vi "1.8.0 Mutation.vi"(8 "error in":errorcluster, 11 "Device Ref in":T1 format="%.0x") -> (0 "error out":errorcluster, 3 "Device Ref out":T1 format="%.0x")   [LabVIEW 2017, in "Ballard Arinc-429 System Explorer.lvlib"]
uses:
  Ballard Arinc-429 System Explorer.lvlib
  <vilib>/NI Veristand/Custom Device API/Custom Device Item Ref.ctl
  <vilib>/NI Veristand/Custom Device Tools/Custom Device Utility Library/Custom Device Utility Library.lvlib
  <vilib>/NI Veristand/Custom Device Tools/Custom Device Utility Library/NI VeriStand - Search for Item by Name.vi
  Shared/Controls and Global/Global.vi
  Shared/Ballard Arinc-429 Shared.lvlib
  <vilib>/NI Veristand/Custom Device API/Custom Device API.lvlib
  NationalInstruments.VeriStand.SystemStorage
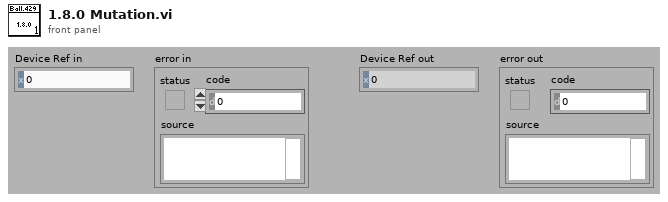
[diagram p1: front panel]
types:
  T1 = typedef "Custom Device API.lvlib/Custom Device Item Ref.ctl" = u64
  T2 = typedef "Custom Device API.lvlib/Custom Device Pointer.ctl" = refnum<k24>
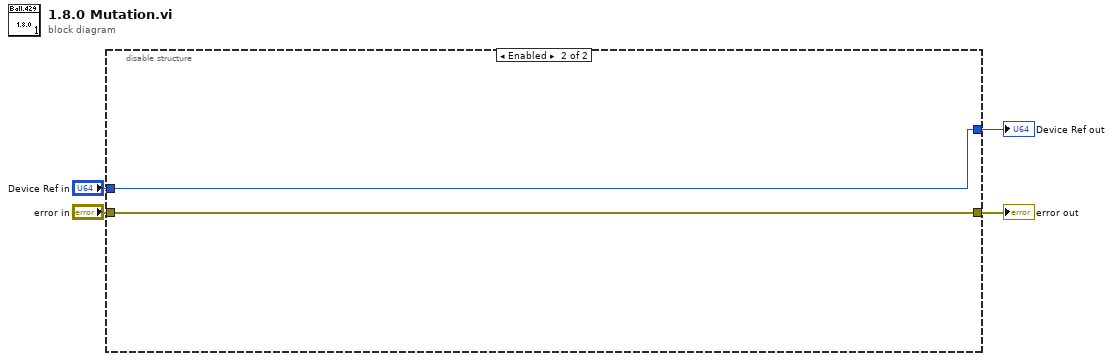
[diagram p0: block diagram]
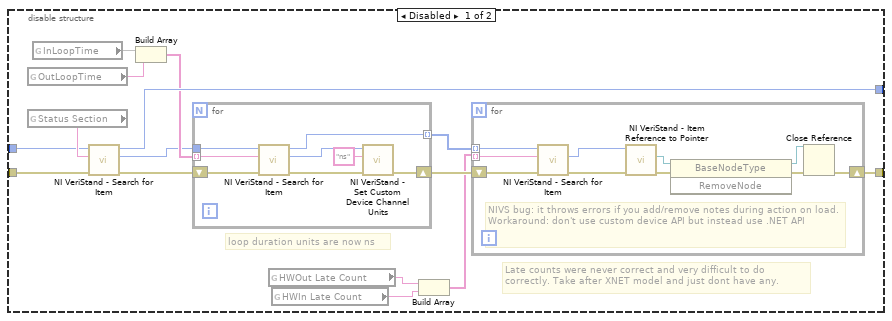
[diagram p2: hidden frame]
diagram:
  n1 = disable-structure shown="Enabled" {
    disable-tunnel: [w19 w39] -> w4
    disable-tunnel: "Device Ref in" -> [w12 w39]
    disable-tunnel: "error in" -> [w11 w38]
    disable-tunnel: [w5 w38] -> w1
    frame Disabled {
      # "Late counts were never correct and very difficult to do correctly. Take after XNET model and just dont have any."
      # "loop duration units are now ns"
      n2 = global read "Global.vi" "OutLoopTime"() -> (w17:string)
      n3 = global read "Global.vi" "Status Section"() -> (w13:string)
      n4 = global read "Global.vi" "InLoopTime"() -> (w16)
      n5 = call-poly <vilib>:"NI VeriStand - Search for Item.vi"("error in"=w11, "Item Name"=w13, "Section Ref in"=w12) -> ("error out"=w15:errorcluster, "Item Ref"=w14:T1, "Section Ref out"=w19:T1)  [unwired: 5 in, 1 out]
      n6 = Build Array(w16, w17) -> (w18:string[])
      n7 = for {
        tunnel: w14 -> [w37]
        shift-right: [w33] -> w9
        shift-left: w15 -> [w36]
        tunnel: w18 -> [w35] mode=indexing
        tunnel: [w30] -> w10 mode=indexing
        n8 = call-poly <vilib>:"NI VeriStand - Search for Item.vi"("error in"=w36, "Item Name"=w35, "Section Ref in"=w37) -> ("error out"=w34:errorcluster, "Item Ref"=w32:T1, "Section Ref out"=w30:T1)  [unwired: 5 in, 1 out]
        n9 = call <vilib>:"NI VeriStand - Set Custom Device Channel Units.vi"("error in (no error)"=w34, "Units"="ns", "Channel Ref in"=w32) -> ("error out"=w33:errorcluster)  [unwired: 7 in, 1 out]
      }
      n10 = global read "Global.vi" "HWOut Late Count"() -> (w8:string)
      n11 = global read "Global.vi" "HWIn Late Count"() -> (w7:string)
      n12 = Build Array(w8, w7) -> (w6:string[])
      n13 = for {
        tunnel: w10 -> [w29] mode=indexing
        shift-right: [w21] -> w5
        shift-left: w9 -> [w28]
        tunnel: w6 -> [w27] mode=indexing
        # "NIVS bug: it throws errors if you add/remove notes during action on load. Workaround: don't use custom device API but instead use .NET API"
        n14 = call-poly <vilib>:"NI VeriStand - Search for Item.vi"("error in"=w28, "Item Name"=w27, "Section Ref in"=w29) -> ("error out"=w26:errorcluster, "Item Ref"=w25:T1)  [unwired: 5 in, 2 out]
        n15 = call <vilib>:"NI VeriStand - Item Reference to Pointer.vi"("error in (no error)"=w26, "Item Ref in"=w25) -> ("error out"=w23:errorcluster, "Node Pointer"=w24:T2)  [unwired: 6 in, 2 out]
        n16 = invoke class="BaseNodeType" method="RemoveNode"(reference=w24, error in=w23) -> (reference out=w20:T2, error out=w22:errorcluster)  [unwired: 1 in, 1 out]
        n17 = Close Reference(reference=w20, error in (no error)=w22) -> (error out=w21:errorcluster)
      }
    }
    frame Enabled {
    }
  }
  "Device Ref out" <- w4
  "error out" <- w1
